vi "GetControlImage.vi"(0 "Control ref":refnum<vi>, 5 "error in (no error)":errorcluster) -> (14 "Image 2":T1, 16 "Image 1":T1, 19 "error out":errorcluster)   [LabVIEW 2014, in "WebFrontPanel.lvclass"]
uses:
  WebFrontPanel.lvclass
  <vilib>/picture/picture.llb/imagedata.ctl
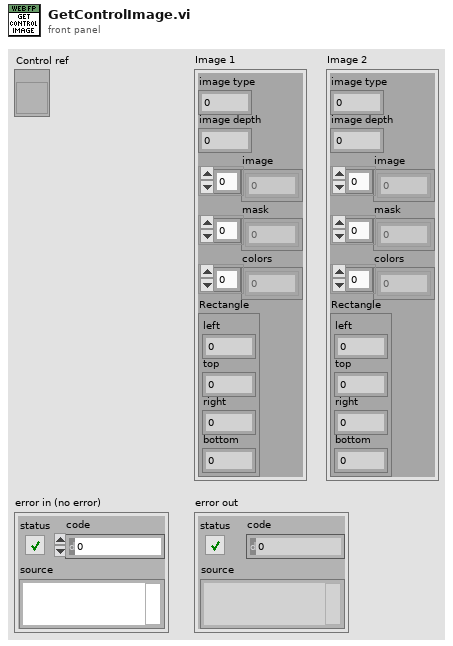
[diagram p1: front panel]
types:
  T1 = typedef "imagedata.ctl" = cluster{"image type":i32, "image depth":i32, "image":u8[], "mask":u8[], "colors":u32[], "Rectangle":cluster{"left":i16, "top":i16, "right":i16, "bottom":i16}}
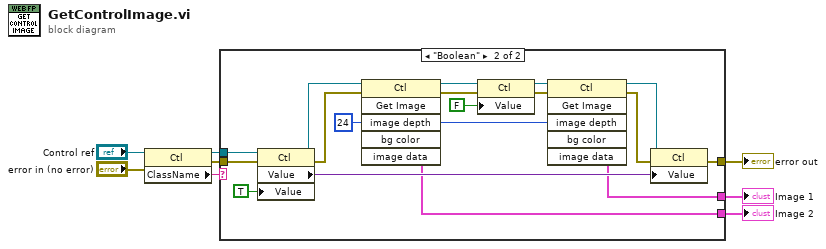
[diagram p0: block diagram]
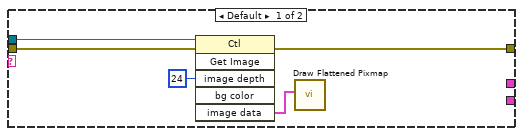
[diagram p2: hidden frame]
diagram:
  n1 = property on="Property Node" class="Ctl"(reference="Control ref", error in="error in (no error)") -> (reference out=w4:refnum<vi>, error out=w2:errorcluster, "ClassName"=w1:string)
  n2 = case shown="\"Boolean\"" w1 {
    tunnel: [_ w14] -> w8
    tunnel: [_ w15] -> w7
    tunnel: [w10 w19] -> w6
    tunnel: w4 -> [w12 w17]
    tunnel: w2 -> [w11 w16]
    frame Default {
      n3 = invoke on="Invoke Node" class="Ctl" method="Get Image"(reference=w12, error in=w11, "image depth"=24 ("Image Depth")) -> (error out=w10:errorcluster, "image data"=w9:T1)  [unwired: 3 in, 4 out]
      n4 = call <vilib>:"Draw Flattened Pixmap.vi"("image data"=w9) -> ()  [unwired: 8 in, 1 out]
    }
    frame "Boolean" {
      w18 = 24 ("Image Depth")
      n5 = property on="Property Node" class="Ctl"(reference=w17, error in=w16, "Value"=TRUE) -> (reference out=w25:refnum<vi>, error out=w22:errorcluster, "Value"=w26:variant)
      n6 = invoke on="Invoke Node" class="Ctl" method="Get Image"(reference=w25, error in=w22, "image depth"=w18) -> (reference out=w24:refnum<vi>, error out=w23:errorcluster, "image data"=w14:T1)  [unwired: 3 in, 3 out]
      n7 = property on="Property Node" class="Ctl"(reference=w24, error in=w23, "Value"=FALSE) -> (reference out=w30:refnum<vi>, error out=w29:errorcluster)
      n8 = invoke on="Invoke Node" class="Ctl" method="Get Image"(reference=w30, error in=w29, "image depth"=w18) -> (reference out=w28:refnum<vi>, error out=w27:errorcluster, "image data"=w15:T1)  [unwired: 3 in, 3 out]
      n9 = property on="Property Node" class="Ctl"(reference=w28, error in=w27, "Value"=w26) -> (error out=w19:errorcluster)  [unwired: 1 out]
    }
  }
  "Image 2" <- w8
  "Image 1" <- w7
  "error out" <- w6
